vi "ClimbOutput.vi"(10 "Driver Right Bumper":bool, 11 "Driver Left Bumper":bool) -> (3 "ClimbOutput":dbl)   [LabVIEW 2018]
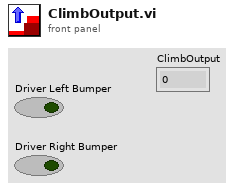
[diagram p1: front panel]
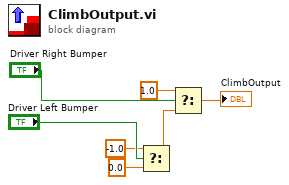
[diagram p0: block diagram]
diagram:
  n1 = Select(t=-1.0, s="Driver Left Bumper", f=0.0) -> (s? t:f=w5:dbl)
  n2 = Select(t=1.0, s="Driver Right Bumper", f=w5) -> (s? t:f=→"ClimbOutput":dbl)
